vi "Stream to AVI Files (Optimized Performance).vi"() -> ()   [LabVIEW 2023]
doc: "The Stream to AVI Files (Optimized Performance) example shows how to save images to an AVI file when using a ring acquisition. This example uses a ring acquisition which is optimized for performance, but has some restrictions on the camera's image format and size. Use the Stream to AVI File example if your camera settings do not work with a ring acquisition."
uses:
  <vilib>/vision/Avi.llb/IMAQ AVI2 Codec Path.ctl
  <vilib>/vision/driver/IMAQdx.llb/IMAQdx Acquisition Mode.ctl
  <vilib>/vision/Image Controls.llb/IMAQ Image.ctl
  <vilib>/vision/driver/IMAQdx.llb/IMAQdx Buffer Number Mode.ctl
  <vilib>/Utility/High Resolution Relative Seconds.vi
  <vilib>/vision/driver/NI_Vision_Acquisition_Software.lvlib
  <resource>/objmgr/imaqdx.rc
panel:
  in  "Skip Count":u32
  out "Images Saved Per Second":dbl
  out "Images Acquired Per Second":dbl
  in  "Images per AVI":i32=100
  out "Write Speed":dbl(graph) caption="Image File Write Speed"
  in  "Start":bool
  in  "Codec":u16(ring) items=["Microsoft Video 1", "Intel IYUV codec", "Cinepak Codec by Radius", "FF Video Codec 1 (FFV1) (NI Vision)", "Motion JPEG (NI Vision)", "Y800 Uncompressed Grey Scale (NI Vision)", "YUV 4:2:0 Planar (NI Vision)"]
  out "Destination Folder":path
  out "Images Behind":i32
  in  "Number of Images":i32=30
  in  "Camera Name":refnum<k21> caption="IMAQdx Session"
  in  "Stop":bool
  # "Overview: Demonstrates how to stream images to an AVI file when using a ring acquisition.\nRequirements: Vision Acquisition Software\nInstructions:\n1. Select the Camera Name\n2. Run the VI\n3. Select the Codec and click Start.\n4. Increase the Skip Count if Images Behind is greater than 0."
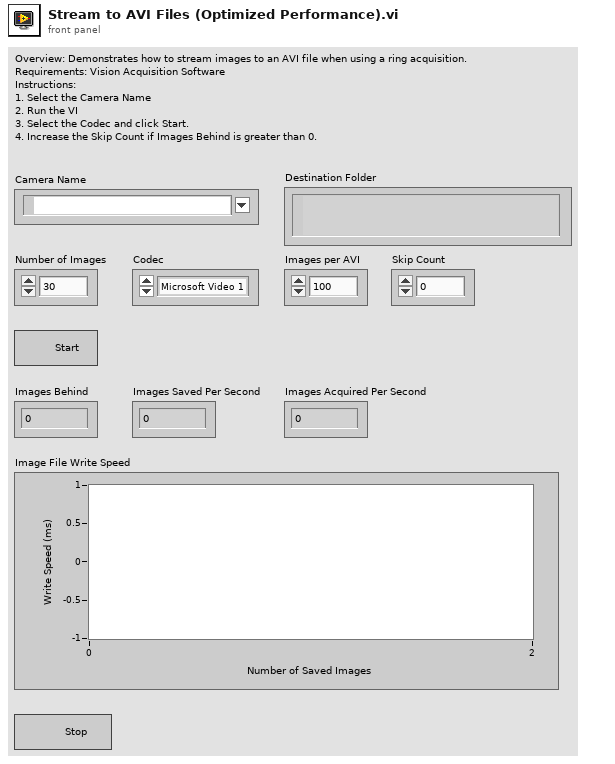
[diagram p1: front panel]
types:
  T1 = typedef "IMAQ AVI2 Codec Path.ctl" = u32
  T2 = typedef "IMAQdx.ctl" = refnum<k21>
  T3 = typedef "IMAQ Image.ctl" = refnum<image>
  T4 = typedef "NI_Vision_Acquisition_Software.lvlib/IMAQdx Acquisition Mode.ctl" = enum32{"One Shot", "Continuous"}
  T5 = typedef "NI_Vision_Acquisition_Software.lvlib/IMAQdx Buffer Number Mode.ctl" = enum32{"Next", "Last", "Buffer Number", "Every", "Last New"}
  T6 = typedef "IMAQ AVI2 Refnum.ctl" = refnum<k20>
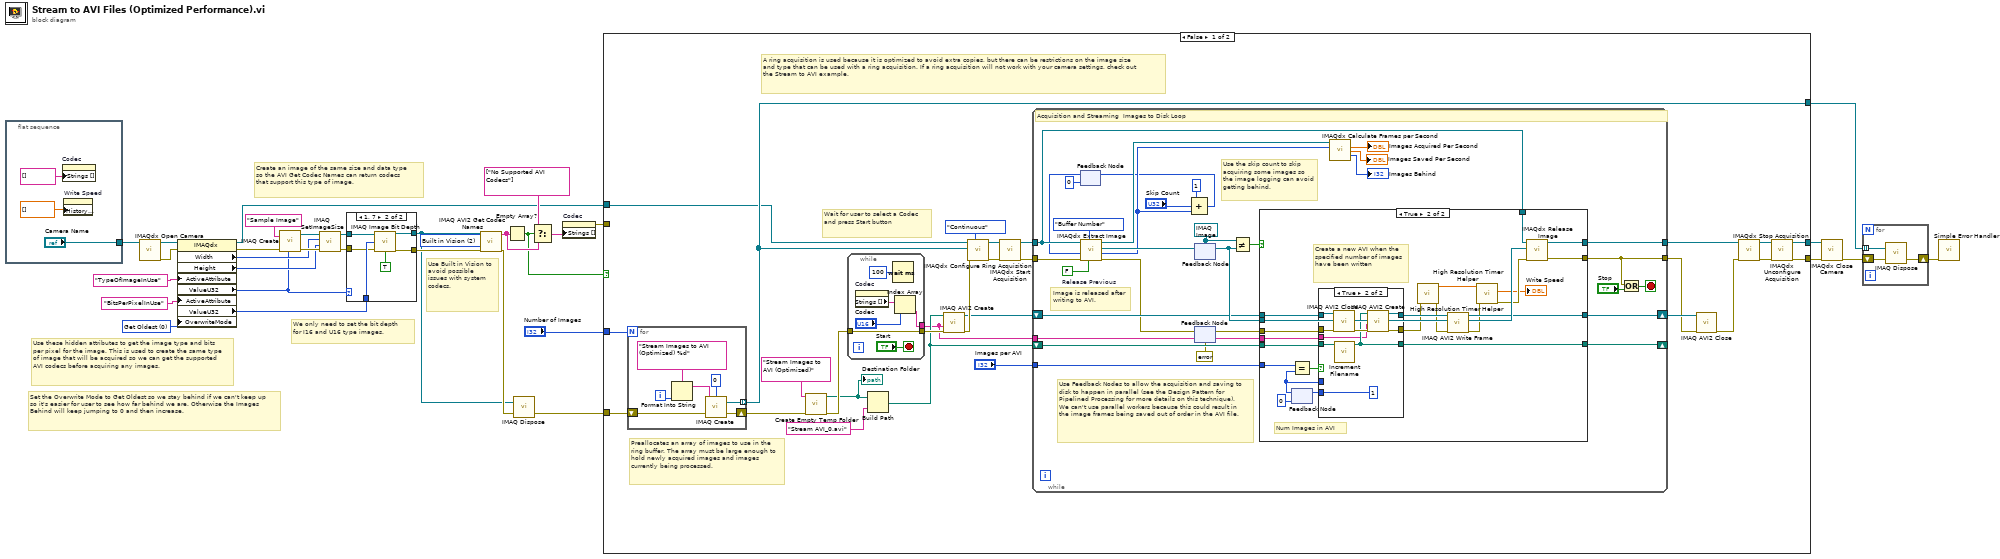
[diagram p0: block diagram]
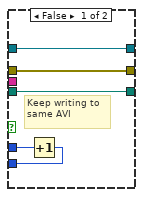
[diagram p4: hidden frame]
diagram:
  w1 = T1 2 items=["Default", "System", "Built in Vision"] ("Codec Source")
  w3 = u32 0 items=["Get Oldest"=0, "Fail"=2, "Get Newest"=3] ("OverwriteMode")
  # "Use Built in Vision to avoid possible issues with system codecs."
  # "Set the Overwrite Mode to Get Oldest so we stay behind if we can't keep up so it's easier for user to see how far behind we are. Otherwise the Images Behind will keep jumping to 0 and then increase."
  # "Create an image of the same size and data type so the AVI Get Codec Names can return codecs that support this type of image."
  # "Use these hidden attributes to get the image type and bits per pixel for the image. This is used to create the same type of image that will be acquired so we can get the supported AVI codecs before acquiring any images."
  # "We only need to set the bit depth for I16 and U16 type images."
  n1 = flat-sequence {
    tunnel: ["Camera Name"] -> w33
    frame #0 {
      n2 = property on="Codec" class="Ring (strict)"("Strings []"=string[] []) -> ()  [unwired: 2 in, 2 out]
      n3 = property on="Write Speed" class="WFChart (strict)"("History Data"=dbl[] []) -> ()  [unwired: 2 in, 2 out]
    }
  }
  n4 = call <vilib>:"IMAQdx Open Camera.vi"("Session In"=w33) -> ("error out"=w27:errorcluster, "Session Out"=w28:T2)  [unwired: 2 in, 7 out]
  n5 = property class="IMAQdx"(reference=w28, error in=w27, "ActiveAttribute"="TypeOfImageInUse", "ActiveAttribute"="BitsPerPixelInUse", "OverwriteMode"=w3) -> (reference out=w12:T2, error out=w25:errorcluster, "Width"=w21:u32, "Height"=w20:u32, "ValueU32"=w7:u32, "ValueU32"=w10:u32)
  n6 = call "IMAQ Create"("Image Name"="Sample Image", "Image Type"=w7, "error in (no error)"=w25) -> ("New Image"=w22:T3, "error out"=w23:errorcluster)  [unwired: 1 in, 1 out]
  n7 = call "IMAQ SetImageSize"("error in (no error)"=w23, "Y Resolution"=w20, "X Resolution"=w21, "Image"=w22) -> ("error out"=w9:errorcluster, "Image Out"=w8:T3)  [unwired: 1 in]
  n8 = case shown="1, 7" w7 {
    tunnel: [w37 w44] -> w13
    tunnel: w10 -> [_ w43]
    tunnel: w9 -> [w37 w42]
    tunnel: w8 -> [w38 w40]
    tunnel: [w38 w39] -> w4
    frame 0, Default {
    }
    frame 1, 7 {
      n9 = call "IMAQ Image Bit Depth"("Image"=w40, "Bit Depth (0)"=w43, "error in (no error)"=w42, "Get/Set Bit Depth? (Set)"=TRUE) -> ("Image Out"=w39:T3, "error out"=w44:errorcluster)  [unwired: 9 in, 1 out]
    }
  }
  n10 = call "IMAQ AVI2 Get Codec Names"("error in (no error)"=w13, "Codec Source"=w1, "Image"=w4) -> ("error out"=w6:errorcluster, "Codec Names"=w18:string[])  [unwired: 7 in]
  n11 = Empty Array?(array=w18) -> (empty?=w14:bool)
  n12 = call "IMAQ Dispose"("Image"=w4, "error in (no error)"=w6) -> ("error out"=w5:errorcluster)  [unwired: 4 in]
  n13 = Select(t=string[] ["No Supported AVI Codecs"], s=w14, f=w18) -> (s? t:f=w16:string[])
  n14 = property on="Codec" class="Ring (strict)"("Strings []"=w16) -> (error out=w15:errorcluster)  [unwired: 2 in, 1 out]
  n15 = case shown="False" w14 {
    tunnel: [w72 w158] -> w32
    tunnel: [w71 w159] -> w31
    tunnel: "Number of Images" -> [w65 _]
    tunnel: [w64 _] -> w29
    tunnel: w12 -> [w58 w159]
    tunnel: w5 -> [w57 w158]
    tunnel: w15 -> [_ _]
    frame False {
      # "Wait for user to select a Codec and press Start button"
      # "A ring acquisition is used because it is optimized to avoid extra copies, but there can be restrictions on the image size and type that can be used with a ring acquisition. If a ring acquisition will not work with your camera settings, check out the Stream to AVI example."
      # "Preallocates an array of images to use in the ring buffer. The array must be large enough to hold newly acquired images and images currently being processed."
      n16 = for {
        N: w65 -> [_]
        tunnel: [w156] -> w64 mode=indexing
        shift-right: [w155] -> w60
        shift-left: w57 -> [w157]
        i -> [w154]
        n17 = Format Into String(format string="Stream Images to AVI (Optimized) %d" ("Image Name"), w154) -> (resulting string=w153:string)  [unwired: 2 in, 1 out]
        n18 = call "IMAQ Create"("Border Size"=0, "Image Name"=w153, "error in (no error)"=w157) -> ("New Image"=w156:T3, "error out"=w155:errorcluster)  [unwired: 1 in, 1 out]
      }
      n19 = call "Create Empty Temp Folder.vi"("error in (no error)"=w60, "Folder Name"="Stream Images to AVI (Optimized)") -> ("error out"=w56:errorcluster, "Empty Temp Folder"=w48:path)  [unwired: 8 in]
      "Destination Folder" <- w48
      n20 = while {
        tunnel: w56 -> [w149]
        tunnel: [w149] -> w55
        tunnel: [w146] -> w45
        stop <- "Start" stop-if-true
        n21 = property on="Codec" class="Ring (strict)"() -> ("Strings []"=w147:string[])  [unwired: 2 in, 2 out]
        n22 = Wait (ms)(milliseconds to wait=u32 100) -> ()  [unwired: 1 out]
        n23 = Index Array(array=w147, index="Codec") -> (element=w146:string)
      }
      n24 = Build Path(base path=w48, name or relative path="Stream AVI_0.avi") -> (appended path=w46:path)
      n25 = call "IMAQ AVI2 Create"("error in (no error)"=w55, "Codec"=w45, "AVI Path"=w46) -> ("error out"=w54:errorcluster, "AVI Refnum"=w49:T6)  [unwired: 7 in]
      n26 = call <vilib>:"IMAQdx Configure Ring Acquisition.vi"("Mode"=IMAQdx_Acquisition_Mode."Continuous" ("Continuous?"), "error in"=w54, "Images"=w64, "Session In"=w58) -> ("error out"=w67:errorcluster, "Session Out"=w68:T2)  [unwired: 5 in, 1 out]
      n27 = call <vilib>:"IMAQdx Start Acquisition.vi"("error in"=w67, "Session In"=w68) -> ("error out"=w61:errorcluster, "Session Out"=w62:T2)  [unwired: 8 out]
      n28 = while {
        tunnel: w61 -> [w103]
        tunnel: w62 -> [w99]
        tunnel: [w100] -> w63
        tunnel: [w88] -> w52
        shift-right: [w101] -> w53
        shift-left: w49 -> [w87]
        tunnel: "Images per AVI" -> [w82]
        shift-right: [w83] -> _
        shift-left: w46 -> [w84]
        tunnel: w45 -> [w85]
        stop <- w90 stop-if-true
        w97 = FALSE  # Release Previous
        w93 = T3 refnum ("Image Out")
        # "Use the skip count to skip acquiring some images so the image logging can avoid getting behind."
        # "Use Feedback Nodes to allow the acquisition and saving to disk to happen in parallel (see the Design Pattern for Pipelined Processing for more details on this technique). We can't use parallel workers because this could result in the image frames being saved out of order in the AVI file."
        # "Image is released after writing to AVI."
        # "Acquisition and Streaming  Images to Disk Loop"
        n29 = feedback #1(u32 0) -> (w80:u32)
        n30 = call <vilib>:"IMAQdx Extract Image.vi"("Release Previous (true)"=w97, "Buffer Number Mode (Next)"=IMAQdx_Buffer_Number_Mode."Buffer Number" ("Buffer Number Mode"), "error in"=w103, "Buffer Number In"=w80, "Session In"=w99) -> ("error out"=w86:errorcluster, "Buffer Number Out"=w78:u32, "Image Out"=w95:T3, "Session Out"=w96:T2)  [unwired: 3 in]
        n31 = Compound Arithmetic op=ADD(u32 1 ("value"), "Skip Count", w78) -> (w75:u32)
        n32 = feedback-in #1(w75) -> ()
        n33 = feedback-in #2(w86) -> ()
        n34 = feedback #2(errorcluster {"status"=FALSE, "code"=0, "source"=""} ("error out")) -> (w94:errorcluster)
        n35 = feedback-in #3(w95) -> ()
        n36 = feedback #3(w93) -> (w91:T3)
        n37 = Not Equal?(x=w93, y=w91) -> (x != y?=w92:bool)
        n38 = case shown="True" w92 {
          tunnel: w87 -> [w105 w121]
          tunnel: w91 -> [_ w115]
          tunnel: w94 -> [w106 w120]
          tunnel: [w105 w126] -> w101
          tunnel: [w107 w129] -> w100
          tunnel: w99 -> [w107 w128]
          tunnel: [w106 w127] -> w88
          tunnel: w85 -> [_ w119]
          tunnel: w84 -> [w104 w118]
          tunnel: [w104 w116] -> w83
          tunnel: w82 -> [_ w114]
          frame False {
            # "First iteration doesn't have valid image for this pipelined stage."
          }
          frame True {
            # "Create a new AVI when the specified number of images have been written"
            # "Num Images in AVI"
            n39 = feedback #4(0) -> (w125:i32)
            n40 = Equal?(x=w114, y=w125) -> (x = y?=w122:bool)
            n41 = case shown="True" w122 {
              tunnel: [w134 1] -> w124
              tunnel: w125 -> [w135 _]
              tunnel: w121 -> [w133 w142]
              tunnel: [w133 w139] -> w117
              tunnel: w118 -> [w131 w143]
              tunnel: w120 -> [w132 w141]
              tunnel: [w132 w138] -> w113
              tunnel: [w131 w137] -> w116
              tunnel: w119 -> [_ w136]
              frame False {
                # "Keep writing to same AVI"
                n42 = Increment(x=w135) -> (x+1=w134:i32)
              }
              frame True {
                n43 = call "IMAQ AVI2 Close"("error in (no error)"=w141, "AVI Refnum"=w142) -> ("error out"=w140:errorcluster)  [unwired: 9 in]
                n44 = call "Increment Filename.vi"("Path In"=w143) -> ("Incremented Path Out"=w137:path)  [unwired: 10 in]
                n45 = call "IMAQ AVI2 Create"("error in (no error)"=w140, "Codec"=w136, "AVI Path"=w137) -> ("error out"=w138:errorcluster, "AVI Refnum"=w139:T6)  [unwired: 7 in]
              }
            }
            n46 = feedback-in #4(w124) -> ()
            n47 = call "High Resolution Timer Helper.vi"("error in (no error)"=w113) -> ("error out"=w112:errorcluster, "Current Time"=w109:dbl)  [unwired: 8 in, 1 out]
            n48 = call "IMAQ AVI2 Write Frame"("error in (no error)"=w112, "Image"=w115, "AVI Refnum"=w117) -> ("error out"=w111:errorcluster, "Image Out (duplicate)"=w130:T3, "AVI Refnum (duplicate)"=w126:T6)  [unwired: 6 in]
            n49 = call "High Resolution Timer Helper.vi"("error in (no error)"=w111, "Previous Time"=w109) -> ("error out"=w110:errorcluster, "Time Difference (ms)"=→"Write Speed":dbl)  [unwired: 7 in, 1 out]
            n50 = call <vilib>:"IMAQdx Release Image.vi"("error in"=w110, "Image"=w130, "Session In"=w128) -> ("error out"=w127:errorcluster, "Session Out"=w129:T2)  [unwired: 7 in]
          }
        }
        n51 = call <vilib>:"IMAQdx Calculate Frames per Second.vi"("Session In"=w96, "Buffer Number"=w78) -> ("Acquired Frames per Second"=→"Images Acquired Per Second":dbl, "Processed Frames per Second"=→"Images Saved Per Second":dbl, "Images Behind"=→"Images Behind":i32)  [unwired: 7 in, 4 out]
        n52 = Or(x=w88, y="Stop") -> (x .or. y?=w90:bool)
      }
      n53 = call "IMAQ AVI2 Close"("error in (no error)"=w52, "AVI Refnum"=w53) -> ("error out"=w51:errorcluster)  [unwired: 9 in]
      n54 = call <vilib>:"IMAQdx Stop Acquisition.vi"("error in"=w51, "Session In"=w63) -> ("error out"=w69:errorcluster, "Session Out"=w70:T2)  [unwired: 8 out]
      n55 = call <vilib>:"IMAQdx Unconfigure Acquisition.vi"("error in"=w69, "Session In"=w70) -> ("error out"=w72:errorcluster, "Session Out"=w71:T2)  [unwired: 8 out]
    }
    frame True {
      # "No valid AVI Codecs for the image size and image type."
    }
  }
  n56 = call <vilib>:"IMAQdx Close Camera.vi"("error in"=w32, "Session In"=w31) -> ("error out"=w19:errorcluster)  [unwired: 9 out]
  n57 = for {
    shift-right: [w161] -> w2
    shift-left: w19 -> [w162]
    tunnel: w29 -> [w160] mode=indexing
    n58 = call "IMAQ Dispose"("Image"=w160, "error in (no error)"=w162) -> ("error out"=w161:errorcluster)  [unwired: 4 in]
  }
  n59 = call <vilib>:"Simple Error Handler.vi"("error in (no error)"=w2) -> ()  [unwired: 4 in, 5 out]
